vi "PXIe-7962_FPGA (Host).vi"() -> ()   [LabVIEW 2014]
uses:
  <vilib>/FPGAPlugInAG/PXIe-7962R/niLvFpga_Open_PXIe-7962R.vi
  <vilib>/rvi/interface/common/dynamic/niFpgaDynamicAddResources.vi
  <vilib>/LabVIEW Targets/FPGA/FlexRIO/CustomFPGAMethods/79XXR_Method_IOModuleStatusImpl.vi
  <vilib>/Utility/error.llb/Error Cluster From Error Code.vi
  <vilib>/rvi/errors/niLvFpgaAdjustHostInterfaceError.vi
  <vilib>/rvi/interface/common/niFpgaWaitOnOcc.vi
  <instrlib>/_niInstr/Streaming/v1/Host/Public/Start Finite Stream.vi
  <instrlib>/_niInstr/Streaming/v1/Host/Public/Wait for Stream.vi
  <vilib>/FPGAPlugInAG/Dynamic/niLvFpga_Close_Dynamic.vi
  <vilib>/rvi/interface/nirviOpenFPGA/nirviOpenFPGA.xnode
  FPGA Bitfiles/MochiFPGAControl_FPGATargetDRAMCL_pxie7962fpga_aK6xGIfk4E0.lvbitx
  <vilib>/rvi/interface/nirviMethod/nirviMethod.xnode
  <vilib>/rvi/interface/nirviReadWriteControl/nirviReadWriteControl.xnode
  <vilib>/rvi/interface/nirviCloseFPGA/nirviCloseFPGA.xnode
  <instrlib>/_niInstr/Streaming/v1/Host/niInstr Streaming v1 Host.lvlib
  <vilib>/rvi/errors/niLvFpgaMergeErrorWithErrorCode.vi
  <vilib>/rvi/interface/Simulation/niFpgaSimulationCallBeginRW.vi
  NiFpgaLv.dll
  <vilib>/FPGAPlugInAG/Dynamic/niLvFpga_ConfigureFifo_Dynamic.vi
  <vilib>/FPGAPlugInAG/Dynamic/niLvFpga_StartFifo_Dynamic.vi
  <vilib>/FPGAPlugInAG/Dynamic/niLvFpga_ReadFifo_Dynamic.vi
panel:
  in  "?":enum32{"AI 0", "All AI"}(tab)
  out "AI 0":dbl[](graph)
  out "All AI":dbl[][](graph)
  in  "Debug":bool
  out "Stream 1 samples transferred":u64
  out "stream 1 error state":bool
  out "stream 1 not ready state":bool
  out "stream 1 cancel state":bool
  out "stream 1 finite transfer state":bool
  out "stream 1  idle state":bool
  out "Bits out DRAM":u64
  out "Bits to DRAM":u64
  out "Bits to bundling FIFO":u64
  out "Bits aquired":u64
  out "Writes to DMA":u64
  out "Writes to DRAM":u64
  out "Writes to bundling FIFO":u64
  out "Samples Aquired":u64
  out "Voltage":dbl[][](array[numeric])
  out "Counts":i16[][](array[numeric])
  out "error out":errorcluster
  out "samples transferred":u64
  in  "stop":bool
  out "Raw DMA readout":u64[](array[numeric])
  in  "num samples":u64=64000
  in  "Go":bool
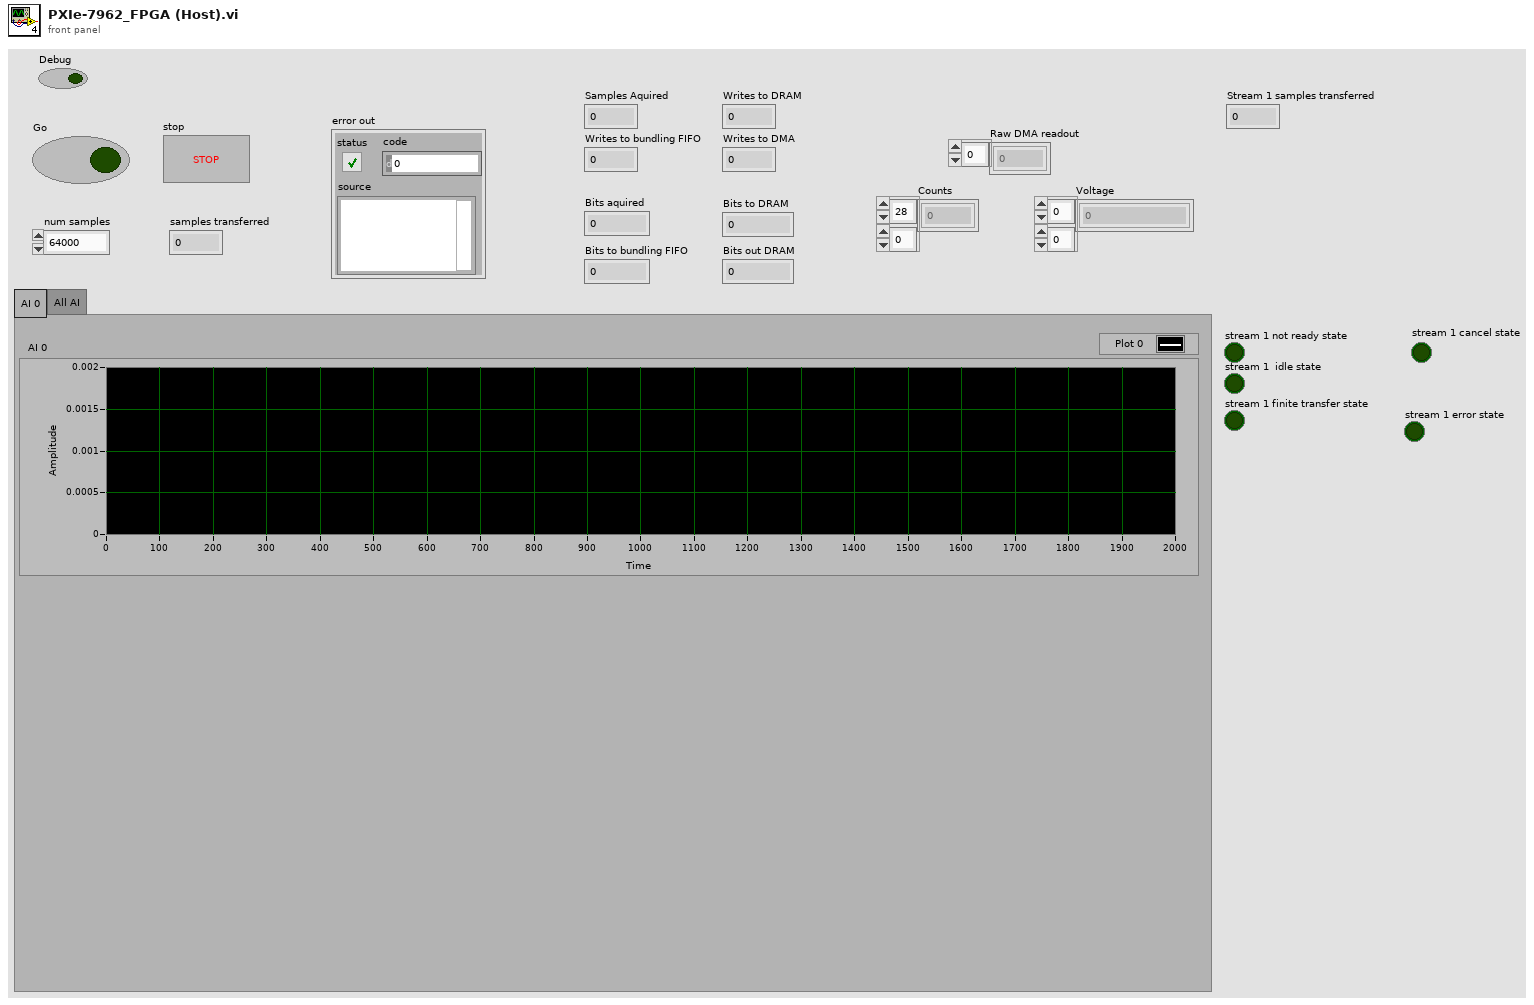
[diagram p1: front panel]
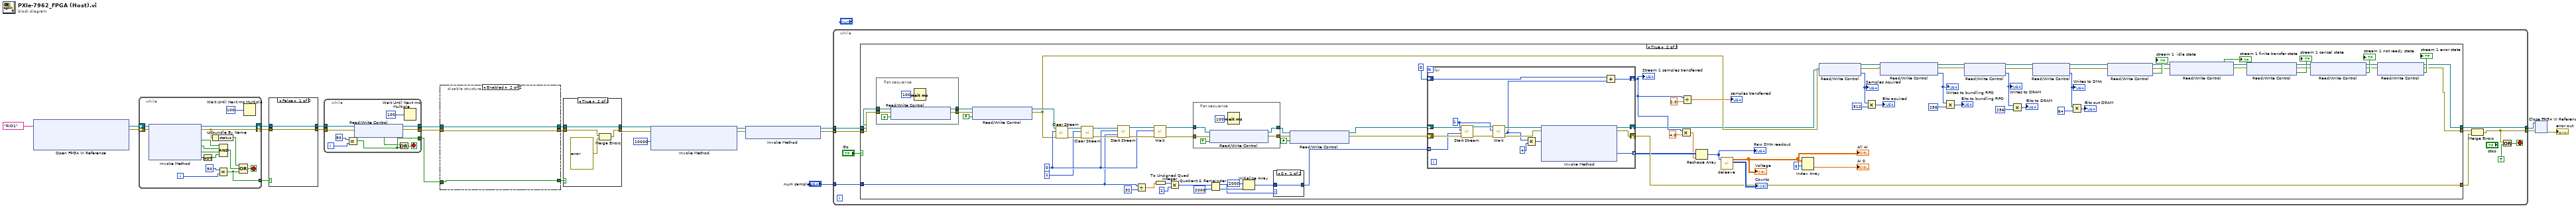
[diagram p0: block diagram]
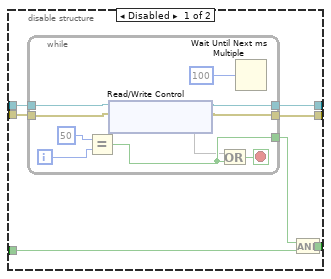
[diagram p2: hidden frame]
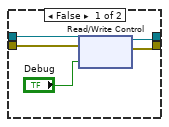
[diagram p3: hidden frame]
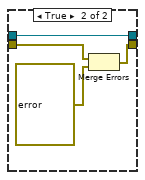
[diagram p4: hidden frame]
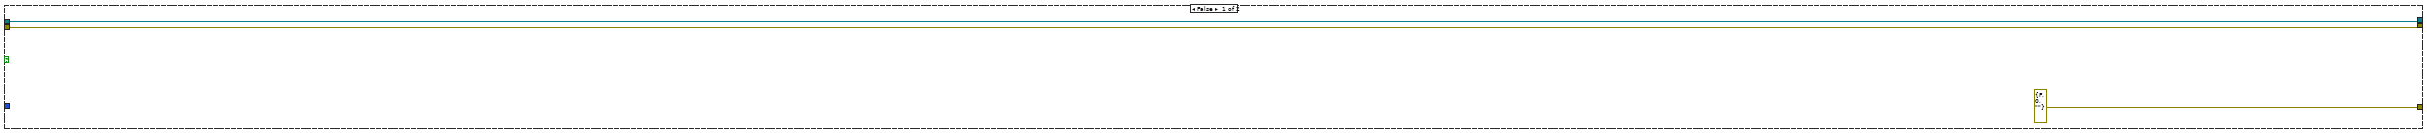
[diagram p5: hidden frame]
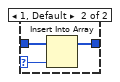
[diagram p6: hidden frame]
diagram:
  n1 = xnode "Open FPGA VI Reference"("resource name"=tag "RIO1") -> ("FPGA VI Reference Out"=w7:refnum<k20>, "error out"=w8:errorcluster)  [unwired: 1 in]
  n2 = while {
    shift-right: [w32] -> w15
    shift-left: w8 -> [w40]
    shift-right: [w39] -> w13
    shift-left: w7 -> [w41]
    tunnel: [w28] -> w14
    i -> [w34]
    stop <- w29 stop-if-true
    n3 = xnode "Invoke Method"("FPGA VI Reference In"=w41, "error in"=w40) -> ("FPGA VI Reference Out"=w39:refnum<k20>, "error out"=w32:errorcluster, "IO Module Present?"=w38:bool, "Power Enabled?"=w37:bool, "IO Enabled?"=w36:bool, "IO Module Mismatch?"=w27:bool)
    n4 = Not(x=w27) -> (.not. x?=w26:bool)
    n5 = Unbundle By Name(w32) -> ("status"=w31:bool)
    n6 = Equal?(x=50, y=w34) -> (x = y?=w28:bool)
    n7 = Compound Arithmetic op=AND(w38, w37, w36, w26) -> (w30:bool)
    n8 = Compound Arithmetic op=OR(w31, w30, w28) -> (w29:bool)
    n9 = Wait Until Next ms Multiple(millisecond multiple=u32 100) -> ()  [unwired: 1 out]
  }
  n10 = case shown="False" w14 {
    tunnel: w15 -> [w42 w46]
    tunnel: [w42 w45] -> w11
    tunnel: w13 -> [w43 w44]
    tunnel: [w43 w44] -> w12
    frame False {
    }
    frame True {
      n11 = Merge Errors(w46, errorcluster {"status"=TRUE, "code"=-1, "source"="The IO Module was not present, powered, or the IO were not enabled.  Verify the NI 5752 is securly connected and try again."} ("error in")) -> (w45:errorcluster)
    }
  }
  n12 = while {
    tunnel: w12 -> [w52]
    tunnel: [w49] -> w6
    tunnel: [w50] -> w5
    tunnel: [w53] -> w3
    tunnel: w11 -> [w51]
    i -> [w56]
    stop <- w54 stop-if-true
    n13 = Equal?(x=50, y=w56) -> (x = y?=w53:bool)
    n14 = xnode "Read/Write Control"("FPGA VI Reference In"=w52, "error in"=w51) -> ("FPGA VI Reference Out"=w49:refnum<k20>, "error out"=w50:errorcluster, "IO Module Init Done"=w48:bool)
    n15 = Or(x=w48, y=w53) -> (x .or. y?=w54:bool)
    n16 = Wait Until Next ms Multiple(millisecond multiple=u32 100) -> ()  [unwired: 1 out]
  }
  n17 = disable-structure shown="Enabled" {
    disable-tunnel: w6 -> [w64 w77]
    disable-tunnel: w5 -> [w63 w76]
    disable-tunnel: [w62 w75] -> w4
    disable-tunnel: w3 -> [w60 w75]
    disable-tunnel: [w59 w77] -> w2
    disable-tunnel: [w58 w76] -> w1
    frame Disabled {
      n18 = while {
        tunnel: w64 -> [w69]
        tunnel: [w66] -> w59
        tunnel: [w67] -> w58
        tunnel: [w70] -> w61
        tunnel: w63 -> [w68]
        i -> [w73]
        stop <- w71 stop-if-true
        n19 = Equal?(x=50, y=w73) -> (x = y?=w70:bool)
        n20 = xnode "Read/Write Control"("FPGA VI Reference In"=w69, "error in"=w68) -> ("FPGA VI Reference Out"=w66:refnum<k20>, "error out"=w67:errorcluster, "DRAM Init Done"=w65)
        n21 = Or(x=w65, y=w70) -> (x .or. y?=w71:bool)
        n22 = Wait Until Next ms Multiple(millisecond multiple=u32 100) -> ()  [unwired: 1 out]
      }
      n23 = And(x=w61, y=w60) -> (x .and. y?=w62:bool)
    }
    frame Enabled {
    }
  }
  n24 = case shown="True" w4 {
    tunnel: w1 -> [w79 w85]
    tunnel: [w78 w84] -> w9
    tunnel: w2 -> [w82 w83]
    tunnel: [w81 w83] -> w10
    frame False {
      n25 = xnode "Read/Write Control"("FPGA VI Reference In"=w82, "error in"=w79, "Debug"="Debug") -> ("FPGA VI Reference Out"=w81:refnum<k20>, "error out"=w78:errorcluster)
    }
    frame True {
      n26 = Merge Errors(w85, errorcluster {"status"=TRUE, "code"=-1, "source"="The IO Module CLIP was not ready. If you are using any external clocks, make sure they are connected and within the supported specifications."} ("error in")) -> (w84:errorcluster)
    }
  }
  n27 = xnode "Invoke Method"("FPGA VI Reference In"=w10, "error in"=w9, "Requested Depth"=u32 10000) -> ("FPGA VI Reference Out"=w24:refnum<k20>, "error out"=w23:errorcluster)  [unwired: 1 out]
  n28 = xnode "Invoke Method"("FPGA VI Reference In"=w24, "error in"=w23) -> ("FPGA VI Reference Out"=w22:refnum<k20>, "error out"=w21:errorcluster)
  n29 = while {
    tunnel: w22 -> [w95]
    tunnel: w21 -> [w94]
    tunnel: "num samples" -> [w93]
    tunnel: [w92] -> w17
    tunnel: [w87] -> w19
    stop <- w91 stop-if-true
    n30 = case shown="True" "Go" {
      tunnel: w95 -> [w99 w124]
      tunnel: w94 -> [w98 w130]
      tunnel: w93 -> [_ w172]
      tunnel: [w98 w119] -> w89
      tunnel: [w99 w118] -> w92
      tunnel: [errorcluster {"status"=FALSE, "code"=0, "source"=""} ("error out") w142] -> w88
      frame False {
      }
      frame True {
        w175 = 0 ("stream index")
        n31 = flat-sequence {
          tunnel: w130 -> [w213]
          tunnel: [w211] -> w128
          tunnel: w124 -> [w210]
          tunnel: [w209] -> w123
          frame #0 {
            n32 = xnode "Read/Write Control"("FPGA VI Reference In"=w210, "error in"=w213, "Reset DRAM write address"=TRUE) -> ("FPGA VI Reference Out"=w209:refnum<k20>, "error out"=w211:errorcluster)
            n33 = Wait (ms)(milliseconds to wait=u32 100) -> ()  [unwired: 1 out]
          }
        }
        n34 = xnode "Read/Write Control"("FPGA VI Reference In"=w123, "error in"=w128, "Reset DRAM write address"=FALSE) -> ("FPGA VI Reference Out"=w122:refnum<k20>, "error out"=w105:errorcluster)
        n35 = call <instrlib>:"Clear Stream.vi"("error in (no error)"=w105, "stream index"=w175, "refnum in"=w122) -> ("error out"=w181:errorcluster, "refnum out"=w182:refnum<k20>)  [unwired: 7 in]
        n36 = call <instrlib>:"Clear Stream.vi"("error in (no error)"=w181, "stream index"=1, "refnum in"=w182) -> ("error out"=w179:errorcluster, "refnum out"=w180:refnum<k20>)  [unwired: 7 in]
        n37 = call-poly <instrlib>:"Start Stream.vi"("error in (no error)"=w179, "num samples"=w172, "stream index"=w175, "refnum in"=w180) -> ("error out"=w176:errorcluster, "refnum out"=w177:refnum<k20>)  [unwired: 6 in]
        n38 = Divide(x=w172, y=u64 32) -> (x/y=w169:dbl)
        n39 = call-poly <instrlib>:"Wait.vi"("error in (no error)"=w176, "stream index"=w175, "refnum in"=w177) -> ("error out"=w125:errorcluster, "refnum out"=w121:refnum<k20>)  [unwired: 5 in, 2 out]
        n40 = To Unsigned Quad Integer(1:w169) -> (0:w170:u64)
        n41 = Multiply(x=w170, y=u64 2) -> (x*y=w111:u64)
        n42 = flat-sequence {
          tunnel: w125 -> [w207]
          tunnel: [w205] -> w126
          tunnel: w121 -> [w204]
          tunnel: [w203] -> w120
          frame #0 {
            n43 = xnode "Read/Write Control"("FPGA VI Reference In"=w204, "error in"=w207, "Reset DRAM read address"=TRUE ("Reset DRAM write address")) -> ("FPGA VI Reference Out"=w203:refnum<k20>, "error out"=w205:errorcluster)
            n44 = Wait (ms)(milliseconds to wait=u32 100) -> ()  [unwired: 1 out]
          }
        }
        n45 = Quotient & Remainder(x=w111, y=u64 2000) -> (x-y*floor(x/y)=w100:u64, floor(x/y)=w109:u64)
        n46 = Initialize Array(u64 2000 ("element"), w109) -> (w107:u64[])
        n47 = case shown="0" w100 {
          selector: w100 -> [_ w184]
          tunnel: w107 -> [w183 w186]
          tunnel: [w183 w185] -> w106
          frame 0 {
          }
          frame 1, Default {
            n48 = Insert Into Array(array=w186, new element=w184) -> (w185:u64[])  [unwired: 1 in]
          }
        }
        n49 = xnode "Read/Write Control"("FPGA VI Reference In"=w120, "error in"=w126, "Reset DRAM read address"=FALSE ("Reset DRAM write address")) -> ("FPGA VI Reference Out"=w112:refnum<k20>, "error out"=w113:errorcluster)
        n50 = for {
          shift-right: [w188] -> w104
          shift-left: w112 -> [w199]
          shift-right: [w187] -> w142
          shift-left: w113 -> [w198]
          shift-right: [w202] -> w115
          shift-left: u64 0 -> [w195]
          tunnel: w106 -> [w196] mode=indexing
          tunnel: [w189] -> w103 mode=indexing
          w197 = 1 ("stream index")
          n51 = call-poly <instrlib>:"Start Stream.vi"("error in (no error)"=w198, "num samples"=w196, "stream index"=w197, "refnum in"=w199) -> ("error out"=w200:errorcluster, "refnum out"=w201:refnum<k20>)  [unwired: 6 in]
          n52 = call-poly <instrlib>:"Wait.vi"("error in (no error)"=w200, "stream index"=w197, "refnum in"=w201) -> ("error out"=w193:errorcluster, "samples transferred"=w191:u64, "refnum out"=w194:refnum<k20>)  [unwired: 5 in, 1 out]
          n53 = Multiply(x=w191, y=u64 4) -> (x*y=w192:u64)
          n54 = xnode "Invoke Method"("FPGA VI Reference In"=w194, "error in"=w193, "Number of Elements"=w192) -> ("FPGA VI Reference Out"=w188:refnum<k20>, "error out"=w187:errorcluster, "Data"=w189:u64[])  [unwired: 1 in, 1 out]
          n55 = Add(x=w195, y=w191) -> (x+y=w202:u64)
        }
        "Stream 1 samples transferred" <- w115
        n56 = Multiply(x=w115, y=4.0) -> (x*y=w102:dbl)
        n57 = Divide(x=w115, y=2.0) -> (x/y=→"samples transferred":dbl)
        n58 = Reshape Array(w103, w102) -> (w101:u64[])
        "Raw DMA readout" <- w101
        n59 = call "deleave.vi"("Data"=w101) -> ("Counts"=→"Counts":i16[][], "Voltage"=w132:dbl[][])  [unwired: 9 in]
        "Voltage" <- w132
        "All AI" <- w132
        n60 = Index Array(array=w132, index (row)=0) -> (element=→"AI 0":dbl[])  [unwired: 1 in]
        n61 = xnode "Read/Write Control"("FPGA VI Reference In"=w104, "error in"=w105) -> ("FPGA VI Reference Out"=w168:refnum<k20>, "error out"=w143:errorcluster, "Samples Aquired"=w164:u64)
        "Samples Aquired" <- w164
        n62 = Multiply(x=w164, y=u64 512) -> (x*y=→"Bits aquired":u64)
        n63 = xnode "Read/Write Control"("FPGA VI Reference In"=w168, "error in"=w143) -> ("FPGA VI Reference Out"=w167:refnum<k20>, "error out"=w141:errorcluster, "Writes to bundeling FIFO"=w160:u64)
        "Writes to bundling FIFO" <- w160
        n64 = Multiply(x=w160, y=u64 256) -> (x*y=→"Bits to bundling FIFO":u64)
        n65 = xnode "Read/Write Control"("FPGA VI Reference In"=w167, "error in"=w141) -> ("FPGA VI Reference Out"=w166:refnum<k20>, "error out"=w140:errorcluster, "Writes to  DRAM"=w157:u64)
        "Writes to DRAM" <- w157
        n66 = Multiply(x=w157, y=u64 256) -> (x*y=→"Bits to DRAM":u64)
        n67 = xnode "Read/Write Control"("FPGA VI Reference In"=w166, "error in"=w140) -> ("FPGA VI Reference Out"=w153:refnum<k20>, "error out"=w139:errorcluster, "Writes to DMA"=w155:u64)
        "Writes to DMA" <- w155
        n68 = Multiply(x=w155, y=u64 64) -> (x*y=→"Bits out DRAM":u64)
        n69 = xnode "Read/Write Control"("FPGA VI Reference In"=w153, "error in"=w139) -> ("FPGA VI Reference Out"=w151:refnum<k20>, "error out"=w138:errorcluster, "stream 1  idle state"=→"stream 1  idle state":bool)
        n70 = xnode "Read/Write Control"("FPGA VI Reference In"=w151, "error in"=w138) -> ("FPGA VI Reference Out"=w149:refnum<k20>, "error out"=w137:errorcluster, "stream 1 finite transfer state"=→"stream 1 finite transfer state":bool)
        n71 = xnode "Read/Write Control"("FPGA VI Reference In"=w149, "error in"=w137) -> ("FPGA VI Reference Out"=w148:refnum<k20>, "error out"=w136:errorcluster, "stream 1 cancel state"=→"stream 1 cancel state":bool)
        n72 = xnode "Read/Write Control"("FPGA VI Reference In"=w148, "error in"=w136) -> ("FPGA VI Reference Out"=w146:refnum<k20>, "error out"=w135:errorcluster, "stream 1 not ready state"=→"stream 1 not ready state":bool)
        n73 = xnode "Read/Write Control"("FPGA VI Reference In"=w146, "error in"=w135) -> ("FPGA VI Reference Out"=w118:refnum<k20>, "error out"=w119:errorcluster, "stream 1 error state"=→"stream 1 error state":bool)
      }
    }
    n74 = Merge Errors(w89, w88) -> (w87:errorcluster)
    n75 = Or(x=w87, y=TRUE) -> (x .or. y?=w91:bool)
  }
  n76 = xnode "Close FPGA VI Reference"("FPGA VI Reference In"=w17, "error in"=w19) -> ("error out"=→"error out":errorcluster)
